vi "SampleMaster for myRIO.vi"() -> ()   [LabVIEW 2012]
doc: "A sample master that can be run on the computer or RIO"
panel:
  out "ms/it":u32(graph)
  out "iteration":i32
  in  "Service call":bool
  in  "Show Web":bool
  in  "Show Node":bool
  out "Answer":string
  in  "LED":bool
  out "LED reply":string
  out "time":string
  out "Status":string
  in  "stop":bool
  # "Instructions:\n1. Run the VI\n2. Verify that you see the correct time.\n3. Press the LED button. You should see the LED reply change.\nIf you are targetting a myRIO, the LED should change as well.\n4. Debug by clicking Show Node and Show Webpage.\n5. See what is being sent back and forth by clicking Show Node and Show Webpage."
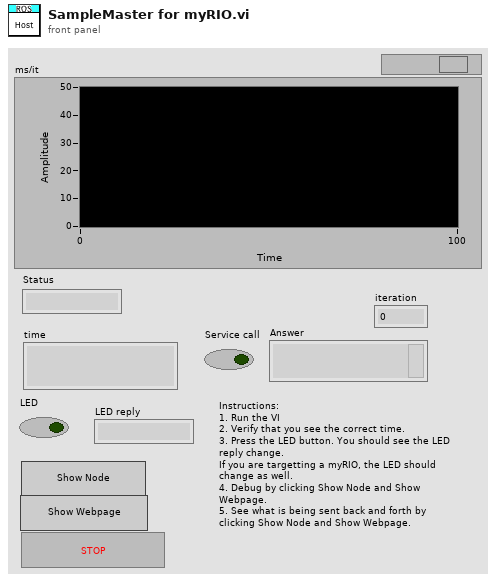
[diagram p1: front panel]
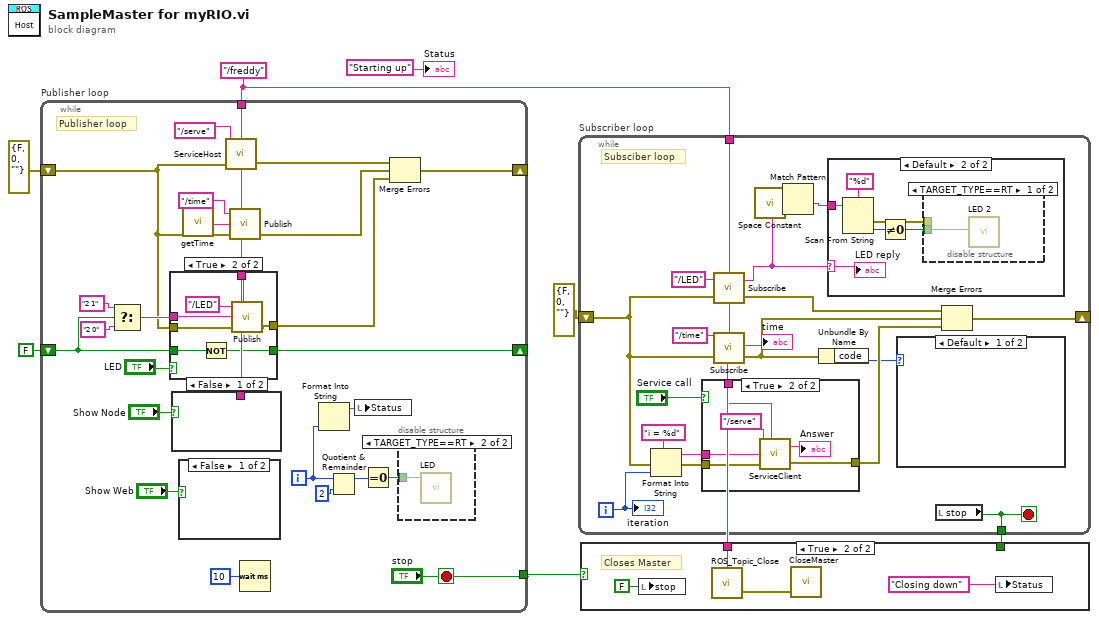
[diagram p0: block diagram]
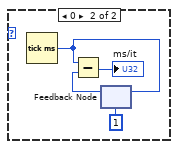
[diagram p2: hidden frame]
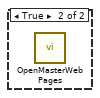
[diagram p8: hidden frame]
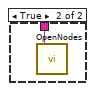
[diagram p10: hidden frame]
diagram:
  w4 = "/freddy" ("Topic")
  n1 = while "Publisher loop" {
    tunnel: ["stop"] -> w5
    tunnel: w4 -> [w19]
    shift-right: [w27] -> _
    shift-left: FALSE -> [w26]
    shift-right: [w12] -> _
    shift-left: errorcluster {"status"=FALSE, "code"=0, "source"=""} ("error out") -> [w10]
    i -> [w15]
    stop <- "stop" stop-if-true
    # "Publisher loop"
    n2 = Select(t="2 1" ("Status"), s=w26, f="2 0" ("Status")) -> (s? t:f=w28:string)
    n3 = case shown="True" "LED" {
      tunnel: w19 -> [_ w38]
      tunnel: w28 -> [_ w37]
      tunnel: [w33 w39] -> w27
      tunnel: w26 -> [w33 w40]
      tunnel: [_ w36] -> w11
      tunnel: w10 -> [_ w34]
      frame False {
      }
      frame True {
        n4 = Not(x=w40) -> (.not. x?=w39:bool)
        n5 = call "Publish.vi"("Topic"="/LED", "node"=w38, "String"=w37, "error in"=w34) -> ("error"=w36:errorcluster)  [unwired: 3 in]
      }
    }
    n6 = case shown="False" "Show Node" {
      tunnel: w19 -> [_ w41]
      frame False {
      }
      frame True {
        n7 = call "OpenNodes.vi"("Node Name"=w41) -> ()  [unwired: 1 in]
      }
    }
    n8 = case shown="False" "Show Web" {
      frame False {
      }
      frame True {
        n9 = call "OpenMasterWebPages.vi"() -> ()  [unwired: 4 in]
      }
    }
    n10 = call "getTime.vi"() -> ("Current Time"=w21:string)  [unwired: 1 in]
    n11 = call "ServiceHost.vi"("error in"=w10, "Topic"="/serve", "node"=w19) -> ("error out"=w14:errorcluster)  [unwired: 1 out]
    n12 = call "Publish.vi"("Topic"="/time", "node"=w19, "String"=w21, "error in"=w10) -> ("error"=w13:errorcluster)  [unwired: 3 in]
    n13 = Wait (ms)(milliseconds to wait=u32 10) -> ()  [unwired: 1 out]
    n14 = Format Into String(w15) -> (resulting string=w31:string)  [unwired: 3 in, 1 out]
    n15 = Quotient & Remainder(x=w15, y=2) -> (x-y*floor(x/y)=w17:i32)  [unwired: 1 out]
    n16 = local write "Status"(w31) -> ()
    n17 = Equal To 0?(x=w17) -> (x = 0?=w16:bool)
    n18 = Merge Errors(w14, w13, w11) -> (w12:errorcluster)
    n19 = disable-structure shown="TARGET_TYPE==RT" {
      disable-tunnel: w16 -> [_ w32]
      frame condition #0 (active) {
      }
      frame condition #1 {
        n20 = call "LED"("LED2"=w32) -> ()  [unwired: 26 in, 1 out]
      }
    }
  }
  n21 = while "Subscriber loop" {
    tunnel: w4 -> [w51]
    shift-right: [w47] -> _
    shift-left: errorcluster {"status"=FALSE, "code"=0, "source"=""} ("error out") -> [w46]
    tunnel: [w48] -> w1
    i -> [w55]
    stop <- w48 stop-if-true
    # "Subsciber loop"
    n22 = Format Into String(format string="i = %d" ("Msg in"), w55) -> (resulting string=w54:string)  [unwired: 2 in, 1 out]
    n23 = case shown="True" "Service call" {
      tunnel: [_ w75] -> w44
      tunnel: w54 -> [_ w74]
      tunnel: w51 -> [_ w73]
      tunnel: w46 -> [_ w72]
      frame False {
      }
      frame True {
        n24 = call "ServiceClient.vi"("Topic"="/serve", "node"=w73, "Msg in"=w74, "error in"=w72) -> ("Reply"=→"Answer":string, "error out"=w75:errorcluster)  [unwired: 1 in]
      }
    }
    n25 = call "Subscribe.vi"("error in"=w46, "Topic"="/LED", "node"=w51) -> ("error out"=w45:errorcluster, "Reply"=w50:string)
    n26 = call "Subscribe.vi"("error in"=w46, "Topic"="/time", "node"=w51) -> ("error out"=w42:errorcluster, "Reply"=→"time":string)
    n27 = call <vilib>:"Space Constant.vi"() -> ("String"=w57:string)
    n28 = Match Pattern(string=w50, regular expression=w57) -> (after substring=w56:string)  [unwired: 1 in, 3 out]
    n29 = Unbundle By Name(w42) -> ("code"=w43:i32)
    n30 = case shown="Default" w50 {
      selector: w50 -> [_ w64]
      tunnel: w56 -> [_ w69]
      frame "" {
      }
      frame Default {
        n31 = Scan From String(format string="%d", input string=w69) -> (error out=w65:errorcluster, output 1=w67:i32)  [unwired: 3 in, 2 out]
        n32 = Not Equal To 0?(x=w67) -> (x != 0?=w66:bool)
        n33 = disable-structure shown="TARGET_TYPE==RT" {
          disable-tunnel: w66 -> [w70 _]
          disable-tunnel: w65 -> [_ _]
          frame condition #0 {
            n34 = call "LED 2"("LED0"=w70) -> ()  [unwired: 26 in, 1 out]
          }
          frame condition #1 (active) {
          }
        }
        "LED reply" <- w64
      }
    }
    n35 = case shown="Default" w43 {
      frame Default {
      }
      frame 0 {
        n36 = Tick Count (ms)() -> (millisecond timer value=w62:u32)
        n37 = feedback-in #1(w62) -> ()
        n38 = feedback #1(u32 1 ("milliseconds to wait")) -> (w61:u32)
        n39 = Subtract(x=w62, y=w61) -> (x-y=→"ms/it":u32)
      }
    }
    n40 = local read "stop"() -> (w48:bool)
    n41 = Merge Errors(w45, w42, w44) -> (w47:errorcluster)
    "iteration" <- w55
  }
  n42 = case shown="True" w5 {
    tunnel: w4 -> [_ w79]
    tunnel: w1 -> [_ _]
    frame False {
    }
    frame True {
      # "Closes Master"
      n43 = local write "stop"(FALSE ("stop")) -> ()
      n44 = call "ROS_Topic_Close.vi"("node"=w79) -> ("error out"=w78:errorcluster)  [unwired: 3 in]
      n45 = call "CloseMaster.vi"("error in (no error)"=w78) -> ()  [unwired: 2 in, 1 out]
      n46 = local write "Status"("Closing down" ("Status")) -> ()
    }
  }
  "Status" <- "Starting up" ("Status")
